vi "heightsensor_1.vi"() -> ()   [LabVIEW 2020]
uses:
  <vilib>/vision/driver/IMAQdx.llb/IMAQdx Buffer Number Mode.ctl
  <vilib>/Utility/file.llb/Write Delimited Spreadsheet (string).vi
  <vilib>/vision/driver/NI_Vision_Acquisition_Software.lvlib
  <vilib>/vision/NI_Vision_Development_Module.lvlib
panel:
  in  "Save  Data?":bool
  in  "Reset":bool
  in  "Flip Camera":bool
  in  "Image Threshold Limits":cluster{sgl, sgl}={128.0, 255.0}
  out "?":bool
  in  "Pumping Rate (µL/min)":dbl format="%#_4g"
  in  "dia (mm)":dbl=16.0 caption="Syringe Diameter" min=0.1 max=50.0
  in  "Syringe COM Port":refnum<visa-resource-name>="COM4"
  out "?":bool
  out "Pump Starting In:":i32(knob) scale=0.0..10.0
  in  "Pump Countdown":i32=10
  out "Need Pump?":bool
  in  "Upper Threshold":dbl=20.0
  in  "Lower Threshold":dbl=-10.0
  out "Height Delta":dbl
  out "Locked Height":dbl
  in  "Lock Height":bool
  out "Average Height":dbl
  out "Current Height":dbl
  out "?":cluster{timestamp[], sgl[]}[](graph)
  in  "Frames Per Average":i32=30
  out "Live Camera View":T1(plugin-control)
  in  "?":bool
  in  "Select Camera":refnum<k21> caption="IMAQdx Session"
  out "Current FPS":dbl
  out "Acquired FPS":dbl
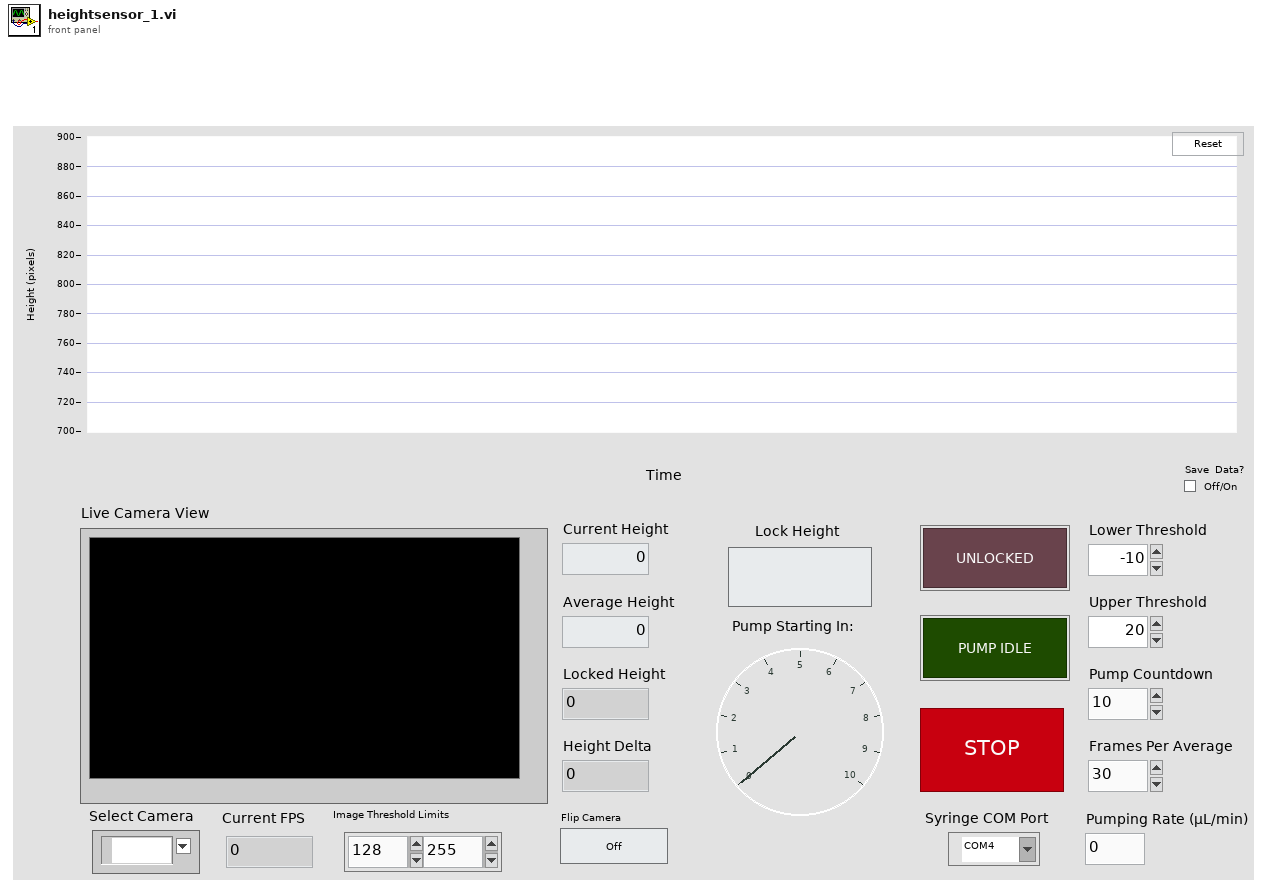
[diagram p1: front panel]
types:
  T1 = typedef "IMAQ Image.ctl" = refnum<image>
  T2 = typedef "IMAQdx.ctl" = refnum<k21>
  T3 = typedef "NI_Vision_Acquisition_Software.lvlib/IMAQdx Buffer Number Mode.ctl" = enum32{"Next", "Last", "Buffer Number", "Every", "Last New"}
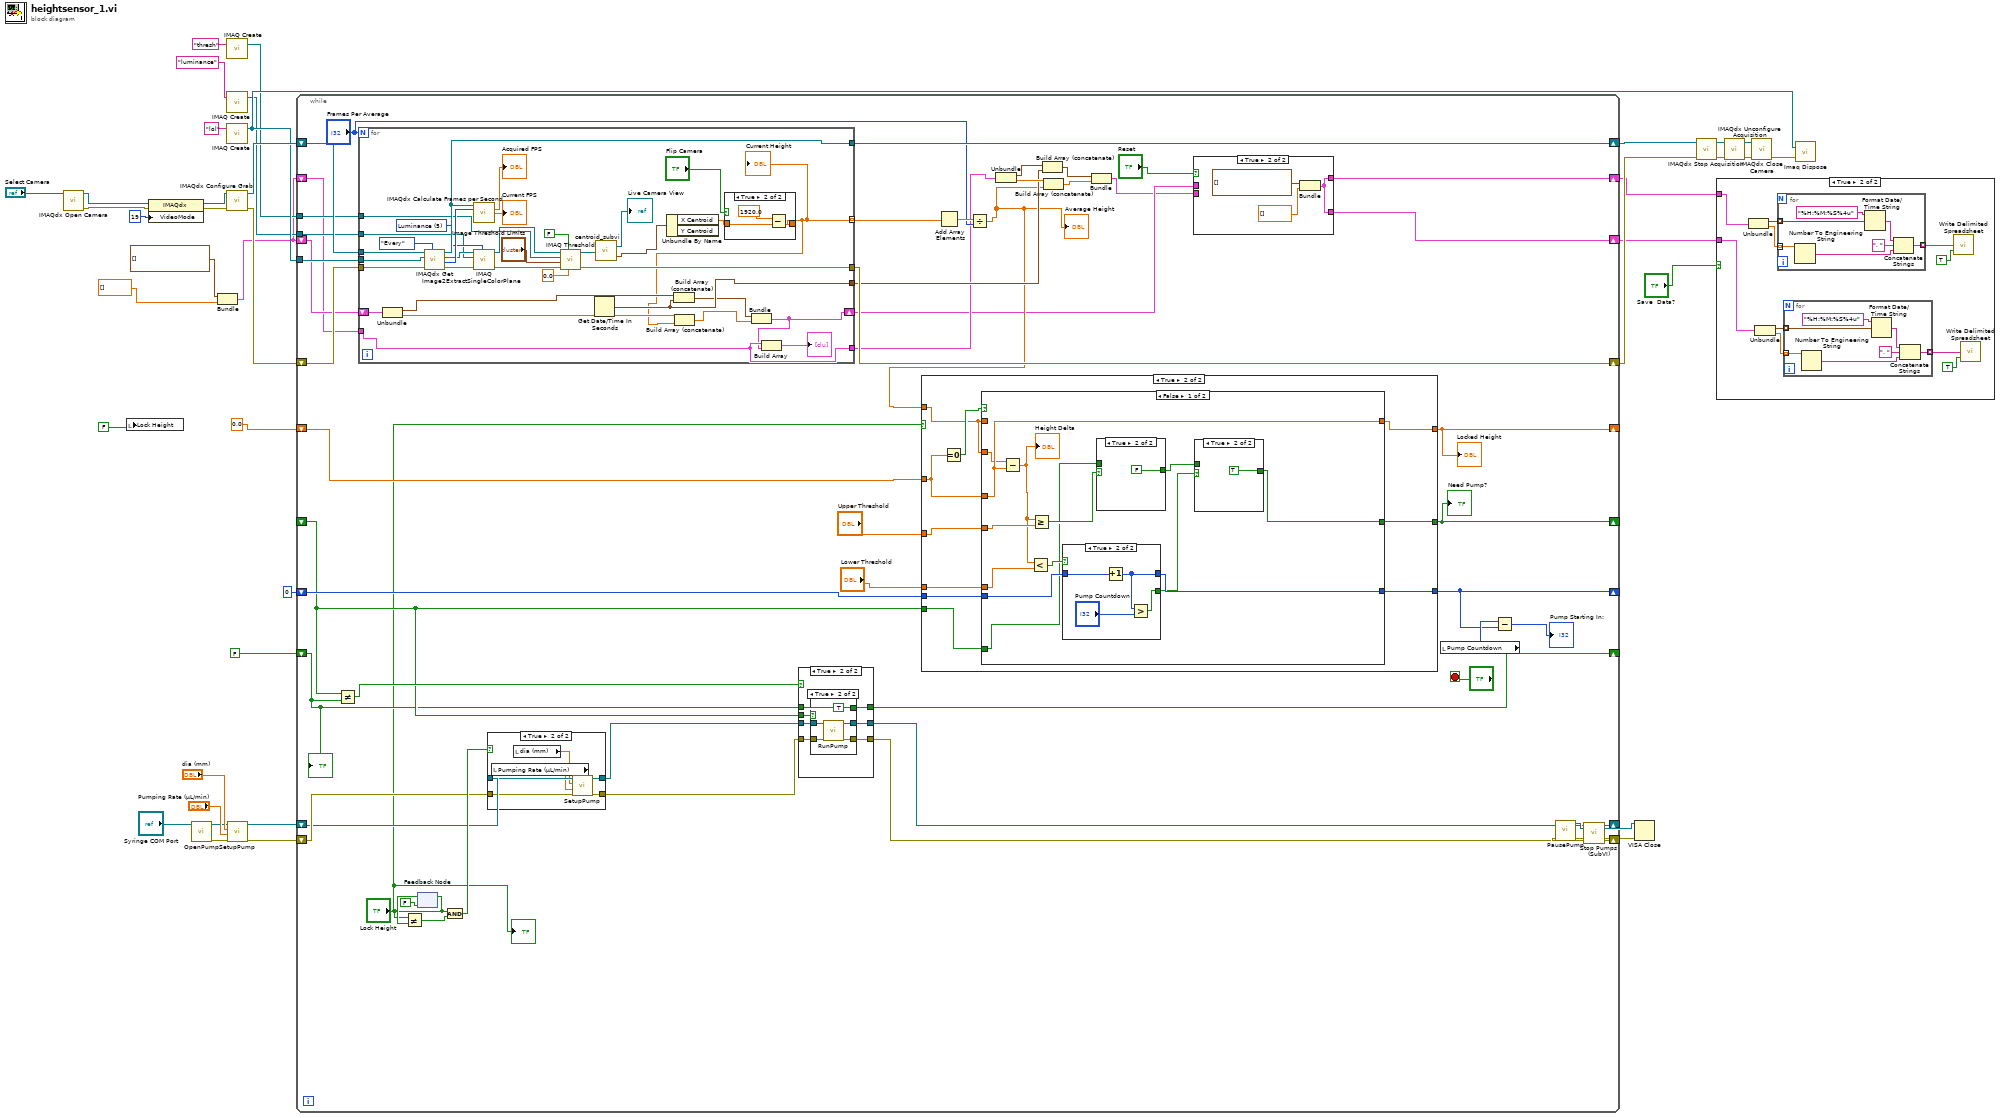
[diagram p0: block diagram]
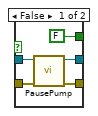
[diagram p6: hidden frame]
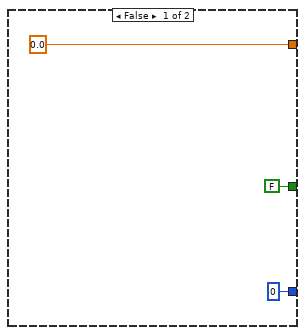
[diagram p7: hidden frame]
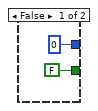
[diagram p10: hidden frame]
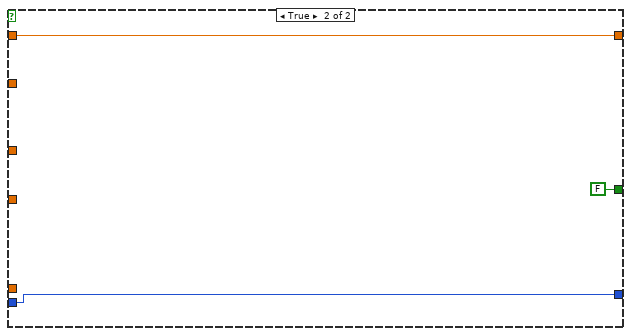
[diagram p11: hidden frame]
diagram:
  n1 = call <vilib>:"IMAQdx Open Camera.vi"("Session In"="Select Camera") -> ("error out"=w30:errorcluster, "Session Out"=w28:T2)  [unwired: 9 in]
  n2 = local write "Lock Height"(FALSE ("Lock")) -> ()
  n3 = property class="IMAQdx"(reference=w28, error in=w30, "VideoMode"=u32 19) -> (reference out=w27:T2, error out=w29:errorcluster)
  n4 = call "OpenPump.vi"("VISA Refnum in"="Syringe COM Port") -> ("error out"=w12:errorcluster, "VISA Refnum out"=w13:refnum<visa-resource-name>)  [unwired: 9 in]
  n5 = Bundle(timestamp[] [], sgl[] []) -> (w21:cluster{timestamp[], sgl[]})  [unwired: 1 in]
  n6 = call "IMAQ Create"("Image Name"="thresh") -> ("New Image"=w24:T1)  [unwired: 4 in, 1 out]
  n7 = call "IMAQ Create"("Image Name"="luminance") -> ("New Image"=w32:T1)  [unwired: 4 in, 1 out]
  n8 = call "IMAQ Create"("Image Name"="lol") -> ("New Image"=w34:T1)  [unwired: 4 in, 1 out]
  n9 = call <vilib>:"IMAQdx Configure Grab.vi"("error in"=w29, "Session In"=w27) -> ("error out"=w43:errorcluster, "Session Out"=w44:T2)  [unwired: 8 in]
  n10 = call "SetupPump.vi"("error in (no error)"=w12, "Set rate"="Pumping Rate (µL/min)", "dia (mm)"="dia (mm)", "VISA Refnum in"=w13) -> ("error out"=w11:errorcluster, "VISA Refnum out"=w10:refnum<visa-resource-name>)  [unwired: 5 in, 1 out]
  n11 = while {
    tunnel: w34 -> [w89]
    tunnel: w32 -> [w88]
    tunnel: w24 -> [w87]
    shift-right: [w91] -> w38
    shift-left: w44 -> [w93]
    shift-right: [w90] -> w37
    shift-left: w43 -> [w92]
    shift-right: [w49] -> w2
    shift-left: w21 -> [w82]
    shift-right: [w47] -> w3
    shift-left: w21 -> [w76]
    shift-right: [w72] -> _
    shift-left: 0.0 -> [w73]
    shift-right: [w52] -> _
    shift-left: 0 -> [w69]
    shift-right: [w68] -> _
    shift-left: _ -> [w66]
    shift-right: [w64] -> _
    shift-left: FALSE -> [w65]
    shift-right: [w63] -> w5
    shift-left: w10 -> [w56]
    shift-right: [w62] -> w4
    shift-left: w11 -> [w57]
    stop <- "?" stop-if-true
    n12 = Not Equal?(x=w66, y=w65) -> (x != y?=w67:bool)
    n13 = for {
      N: "Frames Per Average" -> [_]
      tunnel: w93 -> [w198]
      tunnel: w92 -> [w197]
      tunnel: [w193] -> w91
      tunnel: [w185] -> w90
      tunnel: w89 -> [w194]
      tunnel: w88 -> [w187]
      tunnel: w87 -> [w183]
      tunnel: [w165] -> w84 mode=indexing
      tunnel: [w176] -> w77
      shift-right: [w172] -> w48
      shift-left: w82 -> [w179]
      tunnel: w76 -> [w173]
      tunnel: [w173] -> w75
      w189 = 5 items=["Red", "Green", "Blue", "Hue", "Saturation", "Luminance", "Value", "Intensity"] ("Color Plane")
      n14 = Unbundle(w179) -> (w177:timestamp[], w178:sgl[])
      n15 = call <vilib>:"IMAQdx Get Image2.vi"("Buffer Number Mode (Next)"=IMAQdx_Buffer_Number_Mode."Every" ("Buffer Number Mode"), "error in"=w197, "Image In"=w194, "Session In"=w198) -> ("error out"=w190:errorcluster, "Buffer Number Out"=w192:u32, "Image Out"=w188:T1, "Session Out"=w193:T2)  [unwired: 4 in]
      n16 = call <vilib>:"IMAQdx Calculate Frames per Second.vi"("Session In"=w193, "Buffer Number"=w192) -> ("Acquired Frames per Second"=→"Acquired FPS":dbl, "Processed Frames per Second"=→"Current FPS":dbl)  [unwired: 7 in, 5 out]
      n17 = call "IMAQ ExtractSingleColorPlane"("Color Plane"=w189, "error in (no error)"=w190, "Image Dst"=w187, "Image Src"=w188) -> ("error out"=w186:errorcluster, "Image Dst Out"=w182:T1)  [unwired: 6 in]
      n18 = call "IMAQ Threshold"("Replace Value"=sgl 0.0, "Keep/Replace Value (Replace)"=FALSE, "error in (no error)"=w186, "Range"="Image Threshold Limits", "Image Dst"=w183, "Image Src"=w182) -> ("error out"=w185:errorcluster, "Image Dst Out"=w170:T1)  [unwired: 4 in]
      n19 = Get Date/Time In Seconds() -> (seconds since 1Jan1904=w176:timestamp)
      n20 = call "centroid_subvi.vi"("Refnum in"=w170) -> ("Refnum out"=→"Live Camera View":T1, "Centroid"=w168:cluster{"X Centroid":sgl, "Y Centroid":sgl})
      n21 = Unbundle By Name(w168) -> ("X Centroid"=w166:sgl)  [unwired: 1 out]
      n22 = Build Array (concatenate)(w177, w176) -> (w175:timestamp[])
      n23 = case shown="True" "Flip Camera" {
        tunnel: w166 -> [w199 w201]
        tunnel: [w199 w202] -> w165
        frame False {
        }
        frame True {
          n24 = Subtract(x=sgl 1920.0, y=w201) -> (x-y=w202:sgl)
        }
      }
      "Current Height" <- w165
      n25 = Build Array (concatenate)(w178, w165) -> (w180:sgl[])
      n26 = Bundle(w175, w180) -> (w172:cluster{timestamp[], sgl[]})  [unwired: 1 in]
      n27 = Build Array(w173, w172) -> (→"?":cluster{timestamp[], sgl[]}[])
    }
    n28 = feedback-in #1("Lock Height") -> ()
    n29 = feedback #1(FALSE ("Lock")) -> (w60:bool)
    n30 = Not Equal?(x="Lock Height", y=w60) -> (x != y?=w59:bool)
    n31 = And(x="Lock Height", y=w59) -> (x .and. y?=w58:bool)
    n32 = case shown="True" w58 {
      tunnel: w57 -> [w99 w106]
      tunnel: w56 -> [w100 w105]
      tunnel: [w99 w102] -> w55
      tunnel: [w100 w101] -> w54
      frame False {
      }
      frame True {
        n33 = local read "Pumping Rate (µL/min)"() -> (w104:dbl)
        n34 = local read "dia (mm)"() -> (w103:dbl)
        n35 = call "SetupPump.vi"("error in (no error)"=w106, "Set rate"=w104, "dia (mm)"=w103, "VISA Refnum in"=w105) -> ("error out"=w102:errorcluster, "VISA Refnum out"=w101:refnum<visa-resource-name>)  [unwired: 5 in, 1 out]
      }
    }
    n36 = case shown="True" w67 {
      tunnel: w66 -> [_ w115]
      tunnel: [w109 w114] -> w64
      tunnel: w65 -> [w109 _]
      tunnel: w54 -> [w107 w113]
      tunnel: w55 -> [w108 w112]
      tunnel: [w108 w111] -> w62
      tunnel: [w107 w110] -> w63
      frame False {
      }
      frame True {
        n37 = case shown="True" w115 {
          tunnel: [FALSE TRUE] -> w114
          tunnel: w113 -> [w119 w124]
          tunnel: w112 -> [w118 w123]
          tunnel: [w116 w122] -> w111
          tunnel: [w117 w121] -> w110
          frame False {
            n38 = call "PausePump.vi"("error in (no error)"=w118, "VISA Refnum in"=w119) -> ("error out"=w116:errorcluster, "VISA Refnum out"=w117:refnum<visa-resource-name>)  [unwired: 8 in]
          }
          frame True {
            n39 = call "RunPump.vi"("error in (no error)"=w123, "VISA Refnum in"=w124) -> ("error out"=w122:errorcluster, "VISA Refnum out"=w121:refnum<visa-resource-name>)  [unwired: 8 in]
          }
        }
      }
    }
    n40 = Add Array Elements(numeric array=w84) -> (sum=w85:sgl)
    n41 = Divide(x=w85, y="Frames Per Average") -> (x/y=w74:sgl)
    "Average Height" <- w74
    n42 = case shown="True" "Lock Height" {
      tunnel: w74 -> [_ w135]
      tunnel: w73 -> [_ w136]
      tunnel: [0.0 w137] -> w72
      tunnel: "Upper Threshold" -> [_ w134]
      tunnel: "Lower Threshold" -> [_ w133]
      tunnel: [0 w132] -> w52
      tunnel: w69 -> [_ w131]
      tunnel: [FALSE w130] -> w68
      tunnel: w66 -> [_ w129]
      frame False {
      }
      frame True {
        n43 = Equal To 0?(x=w136) -> (x = 0?=w138:bool)
        n44 = case shown="False" w138 {
          tunnel: w135 -> [_ w164]
          tunnel: [w143 w164] -> w137
          tunnel: w136 -> [w143 _]
          tunnel: w135 -> [w142 _]
          tunnel: w134 -> [w141 _]
          tunnel: w133 -> [w140 _]
          tunnel: [w150 w163] -> w132
          tunnel: w131 -> [w149 w163]
          tunnel: [w144 FALSE] -> w130
          tunnel: w129 -> [w147 _]
          frame False {
            n45 = Subtract(x=w142, y=w143) -> (x-y=w139:dbl)
            "Height Delta" <- w139
            n46 = Less?(x=w139, y=w140) -> (x < y?=w151:bool)
            n47 = Greater Or Equal?(x=w139, y=w141) -> (x >= y?=w148:bool)
            n48 = case shown="True" w151 {
              tunnel: [0 w160] -> w150
              tunnel: w149 -> [_ w161]
              tunnel: [FALSE w158] -> w146
              frame False {
              }
              frame True {
                n49 = Increment(x=w161) -> (x+1=w160:i32)
                n50 = Greater?(x=w160, y="Pump Countdown") -> (0:w158:bool)
              }
            }
            n51 = case shown="True" w148 {
              tunnel: [w154 FALSE] -> w145
              tunnel: w147 -> [w154 _]
              frame False {
              }
              frame True {
              }
            }
            n52 = case shown="True" w146 {
              tunnel: [w152 TRUE] -> w144
              tunnel: w145 -> [w152 _]
              frame False {
              }
              frame True {
              }
            }
          }
          frame True {
          }
        }
      }
    }
    "Locked Height" <- w72
    "Need Pump?" <- w68
    n53 = Unbundle(w75) -> (w79:timestamp[], w78:sgl[])
    n54 = Build Array (concatenate)(w79, w77) -> (w81:timestamp[])
    n55 = Build Array (concatenate)(w78, w74) -> (w80:sgl[])
    n56 = Bundle(w81, w80) -> (w46:cluster{timestamp[], sgl[]})  [unwired: 1 in]
    n57 = case shown="True" "Reset" {
      tunnel: [w95 w96] -> w49
      tunnel: w48 -> [w95 _]
      tunnel: [w94 w96] -> w47
      tunnel: w46 -> [w94 _]
      frame False {
      }
      frame True {
        n58 = Bundle(timestamp[] [], sgl[] []) -> (w96:cluster{timestamp[], sgl[]})  [unwired: 1 in]
      }
    }
    n59 = local read "Pump Countdown"() -> (w53:i32)
    n60 = Subtract(x=w53, y=w52) -> (x-y=→"Pump Starting In:":i32)
    "?" <- w65
    "?" <- "Lock Height"
  }
  n61 = call "PausePump.vi"("error in (no error)"=w4, "VISA Refnum in"=w5) -> ("error out"=w6:errorcluster, "VISA Refnum out"=w7:refnum<visa-resource-name>)  [unwired: 8 in]
  n62 = call "Stop Pumps (SubVI).vi"("error out 2"=w6, "VISA resource name out 2"=w7) -> ("error out"=w8:errorcluster, "VISA resource name out"=w9:refnum<visa-resource-name>)
  n63 = VISA Close(VISA resource name=w9, error in (no error)=w8) -> ()  [unwired: 1 out]
  n64 = call <vilib>:"IMAQdx Stop Acquisition.vi"("error in"=w37, "Session In"=w38) -> ("error out"=w42:errorcluster, "Session Out"=w41:T2)  [unwired: 8 in]
  n65 = case shown="True" "Save  Data?" {
    tunnel: w3 -> [_ w212]
    tunnel: w2 -> [_ w203]
    frame False {
    }
    frame True {
      n66 = Unbundle(w212) -> (w211:timestamp[], w210:sgl[])
      n67 = Unbundle(w203) -> (w204:timestamp[], w205:sgl[])
      n68 = for {
        tunnel: w211 -> [w226] mode=indexing
        tunnel: w210 -> [w224] mode=indexing
        tunnel: [w221] -> w209 mode=indexing
        n69 = Number To Engineering String(4:w224) -> (0:w223:string)  [unwired: 3 in]
        n70 = Format Date/Time String(time format string (%c)="%H:%M:%S%4u", seconds (now)=w226) -> (date/time string=w225:string)  [unwired: 1 in]
        n71 = Concatenate Strings(w225, ", " ("string"), w223) -> (w221:string)
      }
      n72 = for {
        tunnel: w204 -> [w219] mode=indexing
        tunnel: w205 -> [w217] mode=indexing
        tunnel: [w214] -> w206 mode=indexing
        n73 = Number To Engineering String(4:w217) -> (0:w216:string)  [unwired: 3 in]
        n74 = Format Date/Time String(time format string (%c)="%H:%M:%S%4u", seconds (now)=w219) -> (date/time string=w218:string)  [unwired: 1 in]
        n75 = Concatenate Strings(w218, ", " ("string"), w216) -> (w214:string)
      }
      n76 = call-poly <vilib>:"Write Delimited Spreadsheet.vi"("1D data"=w209, "transpose? (no:F)"=TRUE) -> ()  [unwired: 12 in, 2 out]
      n77 = call-poly <vilib>:"Write Delimited Spreadsheet.vi"("1D data"=w206, "transpose? (no:F)"=TRUE) -> ()  [unwired: 12 in, 2 out]
    }
  }
  n78 = call <vilib>:"IMAQdx Unconfigure Acquisition.vi"("error in"=w42, "Session In"=w41) -> ("error out"=w40:errorcluster, "Session Out"=w39:T2)  [unwired: 8 in]
  n79 = call <vilib>:"IMAQdx Close Camera.vi"("error in"=w40, "Session In"=w39) -> ("error out"=w33:errorcluster)  [unwired: 9 in]
  n80 = call "Imaq Dispose"("Image"=w34, "error in (no error)"=w33) -> ()  [unwired: 4 in, 1 out]
